vi "Get Server Debug DLL Path.vi"() -> (0 "DLL Path":path)   [LabVIEW 2019, in "grpc-lvsupport.lvlib"]
uses:
  grpc-lvsupport.lvlib
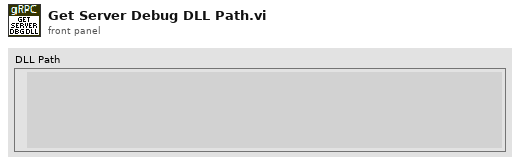
[diagram p1: front panel]
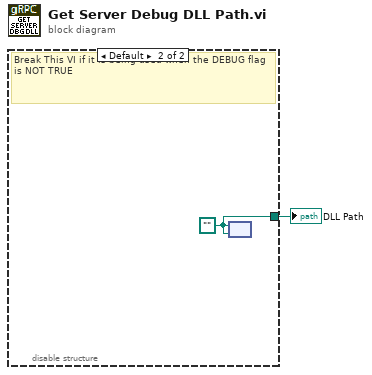
[diagram p0: block diagram]
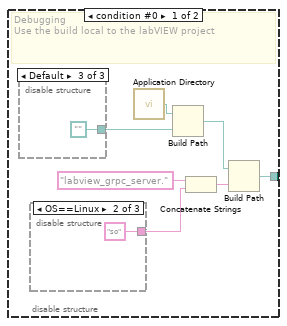
[diagram p2: hidden frame]
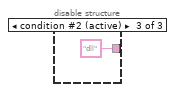
[diagram p4: hidden frame]
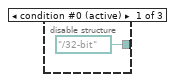
[diagram p5: hidden frame]
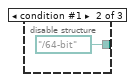
[diagram p6: hidden frame]
diagram:
  n1 = disable-structure shown="Default" {
    disable-tunnel: [w8 w14] -> w1
    frame condition #0 {
      # "Debugging\nUse the build local to the labVIEW project"
      n2 = disable-structure shown="Default" {
        disable-tunnel: [path "../32-bit" path "../64-bit" path ""] -> w2
        frame condition #0 (active) {
        }
        frame condition #1 {
        }
        frame condition #2 {
        }
      }
      n3 = disable-structure shown="OS==Linux" {
        disable-tunnel: [_ "so" "dll"] -> w5
        frame condition #0 {
        }
        frame condition #1 {
        }
        frame condition #2 (active) {
        }
      }
      n4 = call <vilib>:"Application Directory.vi"() -> ("Application Directory"=w6:path)
      n5 = Build Path(base path=w6, name or relative path=w2) -> (appended path=w7:path)
      n6 = Concatenate Strings("labview_grpc_server." ("format string"), w5) -> (w3:string)
      n7 = Build Path(base path=w7, name or relative path=w3) -> (appended path=w8:path)
    }
    frame condition #1 (active) {
      w14 = path ""
      # "Break This VI if it is being used when the DEBUG flag is NOT TRUE"
      n8 = node(w14, w14) -> ()  [unwired: 1 out]
    }
  }
  "DLL Path" <- w1
